vi "main2.0.vi"() -> ()   [LabVIEW 2018]
uses:
  <vilib>/addons/database/Connection.llb/DB Tools Open Connec (Path).vi
  <vilib>/addons/database/NI_Database_API.lvlib
panel:
  out "温度图像":sgl(graph)
  out "负责人信息":T1
  out "疫苗信息":T2 {"生产日期" format="%<%Y/%m/%d>T"}
  in  "CYJ":bool
  in  "比例尺":i16(slide) scale=6.0..18.0
  in  "地图":refnum<k7>(container) caption="网页浏览器"
  out "掉线":bool
  out "经度":string
  out "纬度":string
  out "数据":bool
  in  "stop":bool caption="停止"
  out "时间":timestamp format="%<%x %H:%M:%S>T"
  out "温度":dbl format="%#.1g"
  out "id":i16
  out "定位":bool
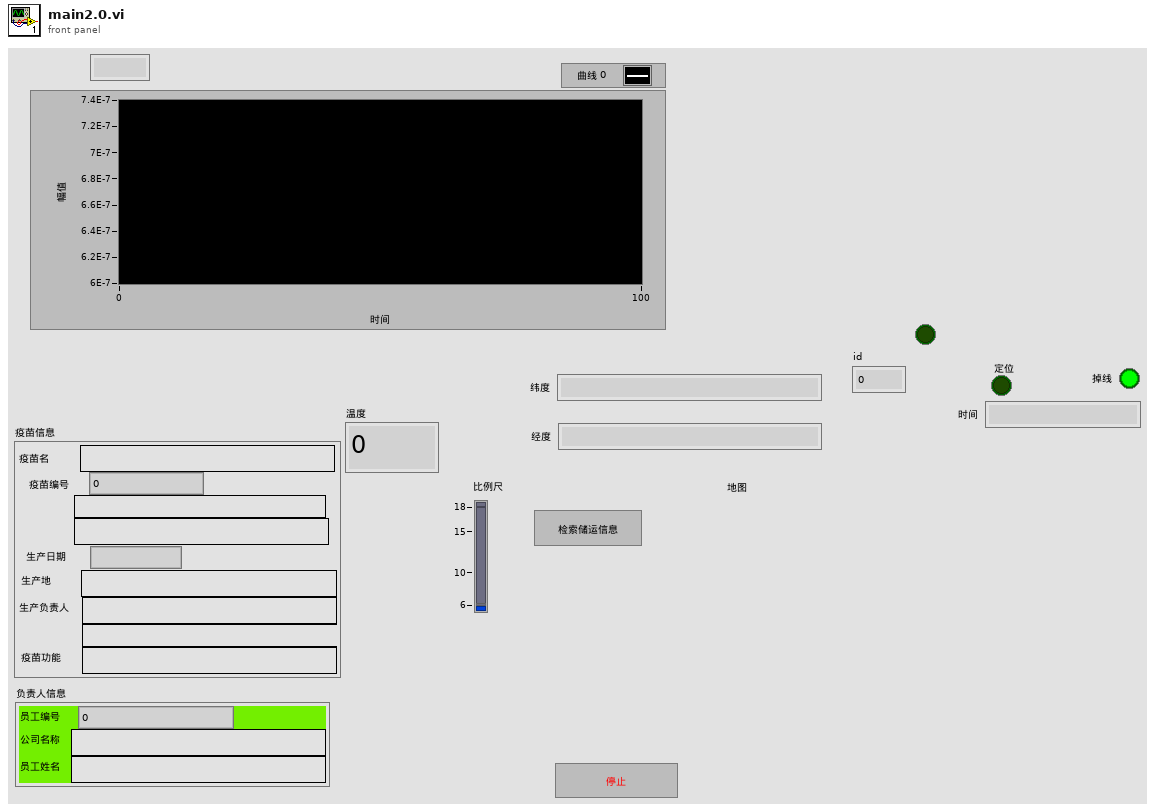
[diagram p1: front panel]
types:
  T1 = typedef "人员信息.ctl" = cluster{"员工编号":i32, "公司名称":string, "员工姓名":string}
  T2 = typedef "疫苗信息.ctl" = cluster{"疫苗名":string, "疫苗编号":i32, "疫苗类型":string, "生产厂家":string, "生产日期":timestamp, "生产地":string, "生产负责人":string, "是否合格":string, "疫苗功能":string}
  T3 = typedef "NI_Database_API.lvlib/Conn ObjectReference.ctl" = refnum<k1>
  T4 = typedef "储运信息.ctl" = cluster{"纬度":sgl, "经度":sgl, "温度":sgl, "负责人":i32, "区域":string, "记录时间":timestamp}
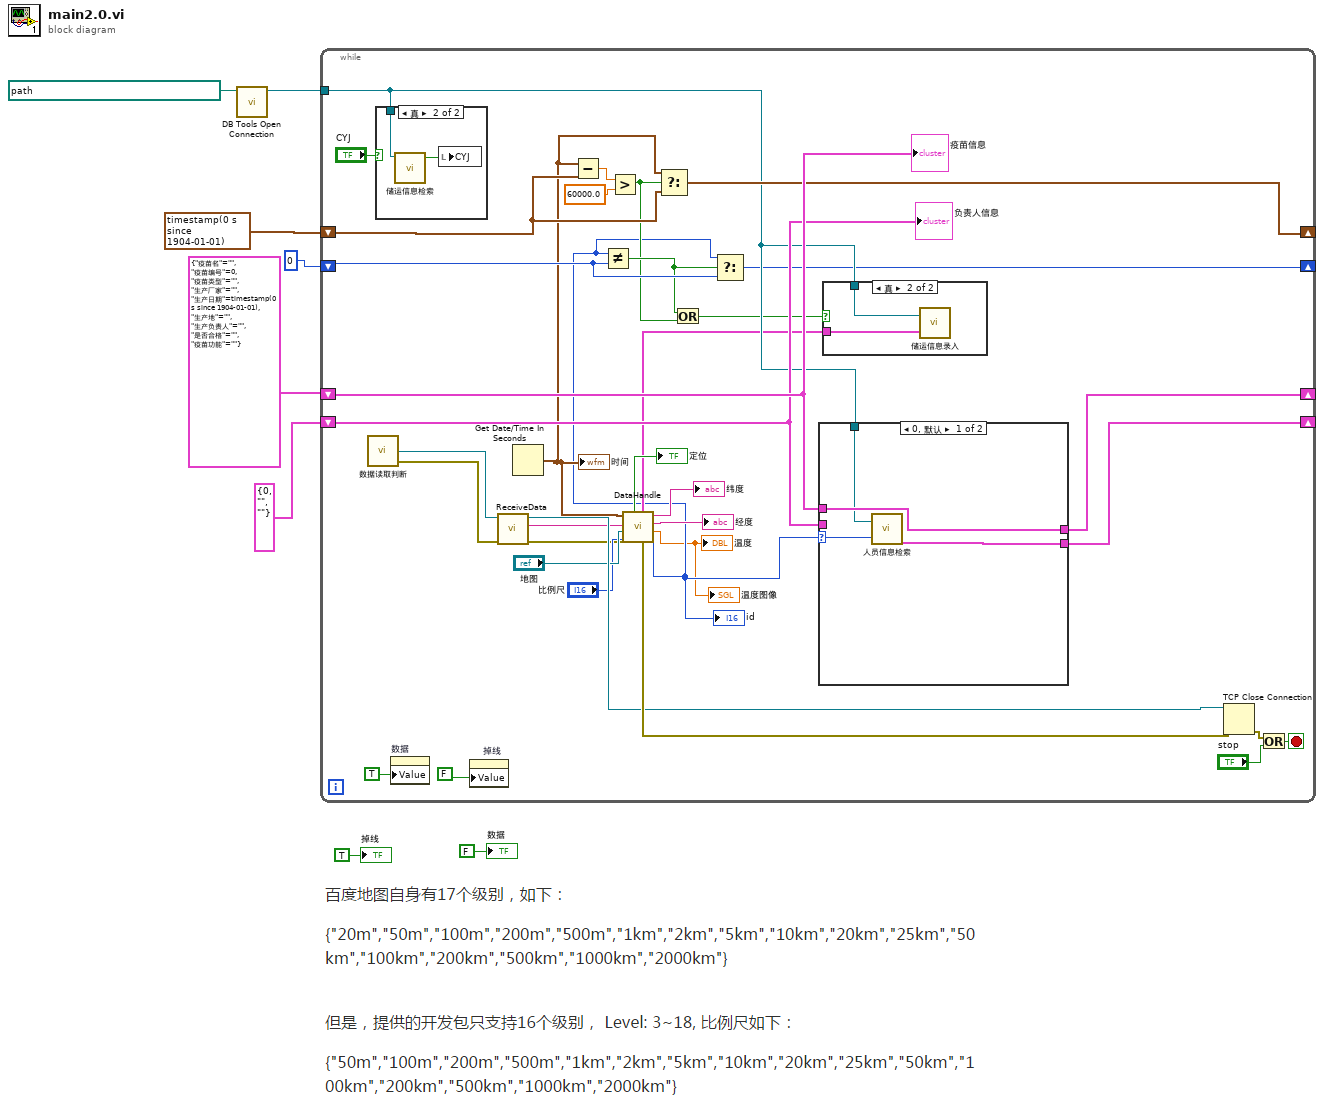
[diagram p0: block diagram]
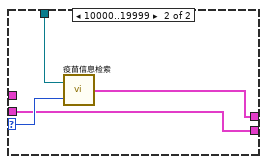
[diagram p3: hidden frame]
diagram:
  n1 = call-poly <vilib>:"DB Tools Open Connection.vi"("connection information"=path "D:/2019毕业设计/Code/GPData.udl" ("路径")) -> ("connection reference"=w6:T3)  [unwired: 7 in, 1 out]
  n2 = while {
    tunnel: w6 -> [w30]
    shift-right: [w29] -> _
    shift-left: T2 {"疫苗名"="", "疫苗编号"=0, "疫苗类型"="", "生产厂家"="", "生产日期"=timestamp(0 s since 1904-01-01), "生产地"="", "生产负责人"="", "是否合格"="", "疫苗功能"=""} ("簇") -> [w35]
    shift-right: [w33] -> _
    shift-left: T1 {"员工编号"=0, "公司名称"="", "员工姓名"=""} ("负责人数据") -> [w34]
    shift-right: [w31] -> _
    shift-left: timestamp(0 s since 1904-01-01) ("时间标识") -> [w32]
    shift-right: [w27] -> _
    shift-left: 0 -> [w28]
    stop <- w43 stop-if-true
    n3 = call "数据读取判断.vi"() -> ("error out"=w40:errorcluster, "connection ID"=w41:refnum<k5>)  [unwired: 1 out]
    n4 = case shown="真" "CYJ" {
      tunnel: w30 -> [_ w55]
      frame False {
      }
      frame True {
        n5 = call "储运信息检索.vi"("connection reference"=w55) -> ("布尔"=w54:bool)  [unwired: 3 in, 2 out]
        n6 = local write "CYJ"(w54) -> ()
      }
    }
    n7 = property on="数据" class="Bool (严格)"("Value"=TRUE ("状态")) -> ()  [unwired: 2 in, 2 out]
    n8 = property on="掉线" class="Bool (严格)"("Value"=FALSE ("掉线")) -> ()  [unwired: 2 in, 2 out]
    n9 = call "ReceiveData.vi"("错误输入（无错误）"=w40, "连接ID"=w41) -> ("错误输出"=w15:errorcluster, "dataOut"=w9:string, "连接ID输出"=w37:refnum<k5>)  [unwired: 5 in, 2 out]
    n10 = Get Date/Time In Seconds() -> (seconds since 1Jan1904=w18:timestamp)
    "时间" <- w18
    n11 = Subtract(x=w18, y=w32) -> (x-y=w24:dbl)
    n12 = Greater?(x=w24, y=60000.0) -> (0:w21:bool)
    n13 = call "DataHandle.vi"("error IO"=w15, "滑动杆"="比例尺", "地图"="地图", "data"=w9, "时间"=w18) -> ("uid"=w11:i16, "温度"=→"温度" →"温度图像":sgl, "经度显示"=→"经度":string, "纬度显示"=→"纬度":string, "错误输出"=w39:errorcluster, "储运信息簇"=w12:T4, "定位"=→"定位":bool)
    "id" <- w11
    n14 = Not Equal?(x=w11, y=w28) -> (x != y?=w22:bool)
    n15 = Select(t=w18, s=w21, f=w32) -> (s? t:f=w31:timestamp)
    n16 = Or(x=w22, y=w21) -> (x .or. y?=w20:bool)
    n17 = Select(t=w11, s=w22, f=w28) -> (s? t:f=w27:i32)
    n18 = case shown="0, 默认" w11 {
      selector: w11 -> [w49 w53]
      tunnel: [w48 w52] -> w29
      tunnel: w35 -> [w48 _]
      tunnel: w34 -> [_ w51]
      tunnel: [w47 w51] -> w33
      tunnel: w30 -> [w46 w50]
      frame 0, Default {
        n19 = call "人员信息检索.vi"("工作人员编号"=w49, "connection reference"=w46) -> ("负责人数据"=w47:T1)  [unwired: 1 out]
      }
      frame 10000..19999 {
        n20 = call "疫苗信息检索.vi"("疫苗编号"=w53, "connection reference"=w50) -> ("疫苗数据"=w52:T2)
      }
    }
    n21 = case shown="真" w20 {
      tunnel: w30 -> [_ w45]
      tunnel: w12 -> [_ w44]
      frame False {
      }
      frame True {
        n22 = call "储运信息录入.vi"("簇"=w44, "connection reference"=w45) -> ()  [unwired: 1 out]
      }
    }
    n23 = TCP Close Connection(connection ID=w37, error in (no error)=w39) -> (error out=w42:errorcluster)  [unwired: 1 in, 1 out]
    n24 = Or(x=w42, y="stop") -> (x .or. y?=w43:bool)
    "疫苗信息" <- w35
    "负责人信息" <- w34
  }
  "掉线" <- TRUE ("掉线")
  "数据" <- FALSE ("串口")
